vi "DB Tools Drop Table.vi"(6 "error in (no error)":errorcluster, 8 "table":string, 9 "connection reference":T1) -> (0 "error out":errorcluster, 3 "connection reference out":T1)   [LabVIEW 2013, in "NI_Database_API_64.lvlib"]
doc: "Deletes the specified <B>table</B> from the database identified by <B>connection reference</B>."
uses:
  NI_Database_API_64.lvlib
  Connection.llb/Conn ObjectReference.ctl
  Connection.llb/Conn Execute.vi
  Recordset.llb/Rec Destroy - Connection.vi
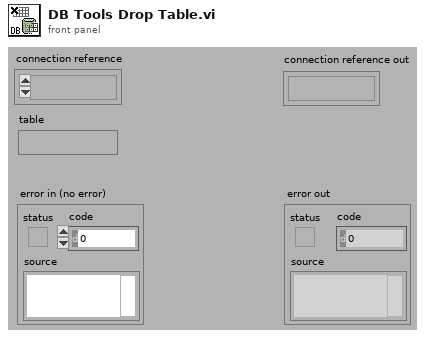
[diagram p1: front panel]
types:
  T1 = typedef "NI_Database_API_64.lvlib/Conn ObjectReference.ctl" = refnum<k1>
  T2 = typedef "NI_Database_API_64.lvlib/Rec ObjectReference.ctl" = refnum<k1>
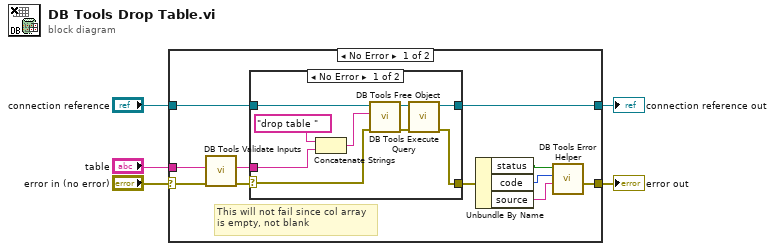
[diagram p0: block diagram]
diagram:
  n1 = case shown="No Error" "error in (no error)" {
    selector: "error in (no error)" -> [w6 w29]
    tunnel: "table" -> [w16 _]
    tunnel: "connection reference" -> [w13 w28]
    tunnel: [w12 w28] -> w3
    tunnel: [w9 w29] -> w2
    frame No Error {
      # "This will not fail since col array\nis empty, not blank"
      n2 = call "DB Tools Validate Inputs.vi"("error in (no error)"=w6, "table"=w16) -> ("error out"=w15:errorcluster, "table out"=w14:string)  [unwired: 3 in, 1 out]
      n3 = case shown="No Error" w15 {
        selector: w15 -> [w20 w26]
        tunnel: w14 -> [w21 _]
        tunnel: w13 -> [w23 w27]
        tunnel: [w17 w26] -> w10
        tunnel: [w19 w27] -> w12
        frame No Error {
          n4 = Concatenate Strings("drop table ", w21) -> (w18:string)
          n5 = call-poly "DB Tools Execute Query.vi"("error in (no error)"=w20, "SQL query"=w18, "connection reference"=w23) -> ("error out"=w24:errorcluster, "recordset reference"=w25:T2)  [unwired: 5 in]
          n6 = call-poly "DB Tools Free Object.vi"("error in (no error)"=w24, "recordset reference"=w25) -> ("error out"=w17:errorcluster, "connection reference"=w19:T1)  [unwired: 8 in]
        }
        frame Error {
        }
      }
      n7 = Unbundle By Name(w10) -> ("status"=w8:bool, "code"=w7:i32, "source"=w11:string)
      n8 = call "DB Tools Error Helper.vi"("source"=w11, "code"=w7, "status"=w8) -> ("error out"=w9:errorcluster)  [unwired: 8 in]
    }
    frame Error {
    }
  }
  "connection reference out" <- w3
  "error out" <- w2
